vi "DAQ_Configure.vi"(8 "error in":errorcluster caption="entrée d'erreur", 10 "Dwell time (µs)":dbl, 11 "Scanning positions":dbl[][](array[numeric])) -> (0 "error out":errorcluster caption="sortie d'erreur", 3 "Task cluster":T1)   [LabVIEW 2026]
uses:
  <vilib>/DAQmx/write.llb/DAQmx Write (Analog 2D DBL NChan NSamp).vi
  <vilib>/DAQmx/create/channels.llb/DAQmx Create Channel (CO-Pulse Generation-Frequency).vi
  <vilib>/DAQmx/configure/timing.llb/DAQmx Timing (Implicit).vi
  <vilib>/DAQmx/create/channels.llb/DAQmx Create Channel (AO-Voltage-Basic).vi
  <vilib>/DAQmx/configure/timing.llb/DAQmx Timing (Sample Clock).vi
  <vilib>/DAQmx/miscellaneous.llb/DAQmx Fill In Error Info.vi
  <vilib>/DAQmx/create/channels.llb/DAQmx Create Channel (AI-Voltage-Basic).vi
  <vilib>/DAQmx/configure/trigger.llb/DAQmx Start Trigger (Digital Edge).vi
  <vilib>/DAQmx/create/channels.llb/DAQmx Create Channel (CI-Pulse Width).vi
  <resource>/objmgr/daqmx.rc
panel:
  out "N samples":u16
  out "Pixel_Freq":dbl
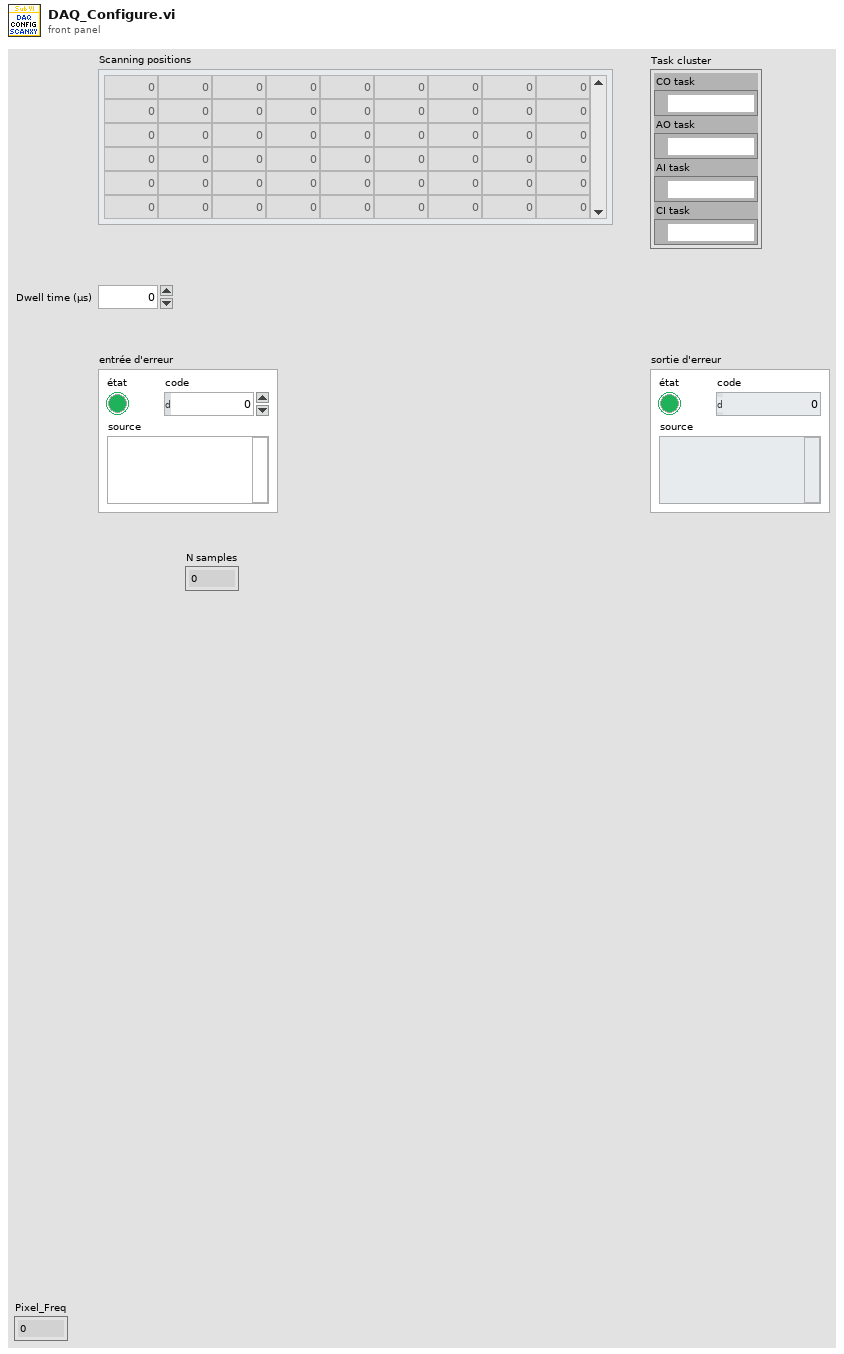
[diagram p1: front panel]
types:
  T1 = cluster{"CO task":refnum<k21>, "AO task":refnum<k21>, "AI task":refnum<k21>, "CI task":refnum<k21>}
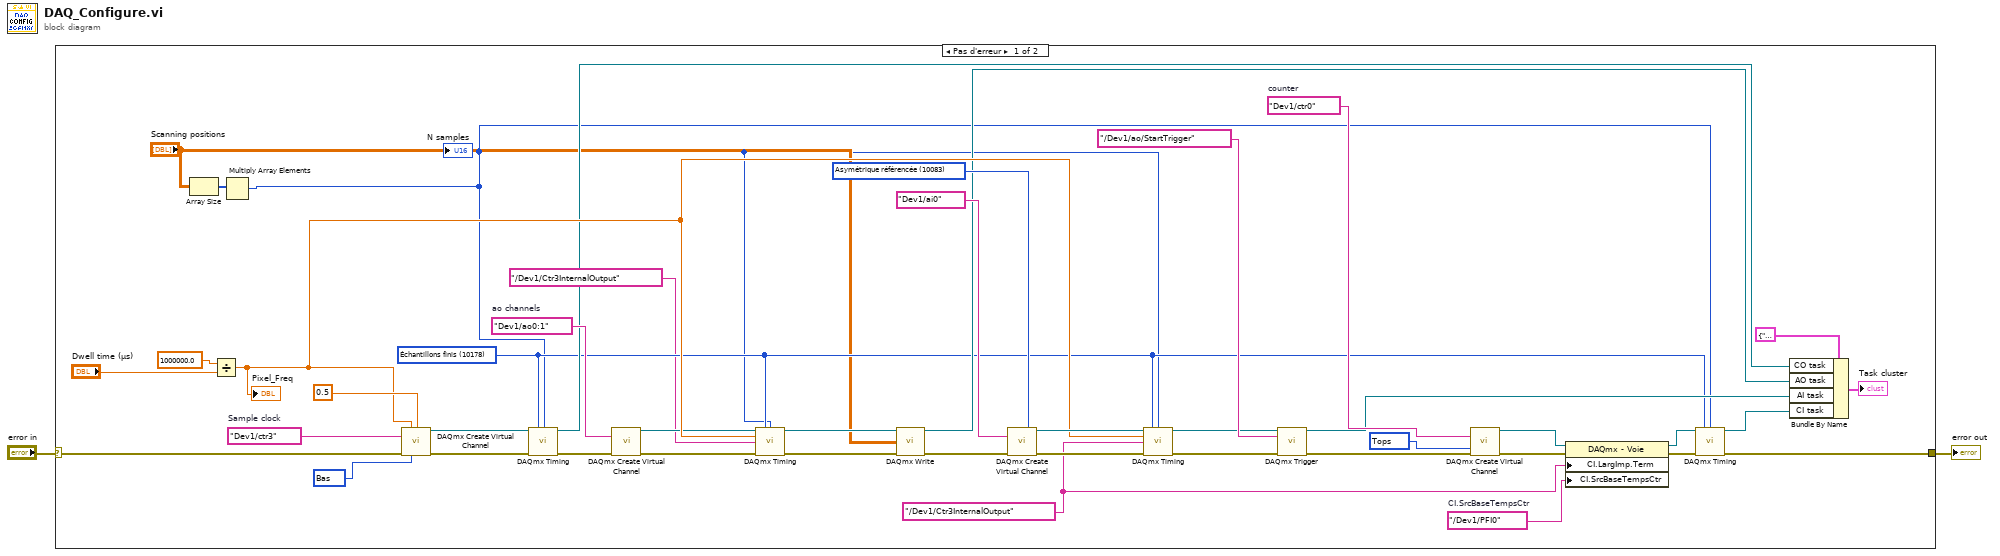
[diagram p0: block diagram]
diagram:
  n1 = case shown="Pas d'erreur" "error in" {
    selector: "error in" -> [w44 w47]
    tunnel: [w13 w47] -> w1
    frame No Error {
      w22 = tag "/Dev1/PFI0"  # CI.SrcBaseTempsCtr
      w28 = 10304 items=["Secondes"=10364, "Tops"=10304, "D'une échelle personnalisée"=10065] ("units")
      w29 = tag "Dev1/ctr0"  # counter
      w25 = tag "/Dev1/Ctr3InternalOutput" ("source")
      w35 = 10083 items=["Par défaut"=-1, "Asymétrique référencée"=10083, "Asymétrique non référencée"=10078, "Différentielle"=10106, "Pseudodifférentielle"=12529] ("input terminal configuration")
      w37 = tag "Dev1/ao0:1"  # ao channels
      w12 = 10178 items=["Échantillons finis"=10178, "Échantillons continus"=10123, "Point par point avec cadencement matériel"=12522] ("sample mode")
      w39 = 10214 items=["Haut"=10192, "Bas"=10214] ("idle state")
      w41 = tag "Dev1/ctr3"  # Sample clock
      n2 = Array Size(array="Scanning positions") -> (size(s)=w5:i32[])
      n3 = Divide(x=1000000.0, y="Dwell time (µs)") -> (x/y=w32:dbl)
      "Pixel_Freq" <- w32
      n4 = Multiply Array Elements(1:w5) -> (0:w3:i32)
      "N samples" <- w3
      n5 = call-poly <vilib>:"DAQmx Create Virtual Channel.vi"("frequency"=w32, "duty cycle"=0.5 ("Duty cycle"), "counter"=w41, "error in"=w44, "idle state"=w39) -> ("task out"=w43:refnum<k21>, "error out"=w42:errorcluster)  [unwired: 9 in]
      n6 = call-poly <vilib>:"DAQmx Timing.vi"("task/channels in"=w43, "sample mode"=w12, "samples per channel"=w3, "error in"=w42) -> ("task out"=w21:refnum<k21>, "error out"=w38:errorcluster)  [unwired: 10 in]
      n7 = call-poly <vilib>:"DAQmx Create Virtual Channel.vi"("physical channels"=w37, "error in"=w38) -> ("task out"=w10:refnum<k21>, "error out"=w11:errorcluster)  [unwired: 12 in]
      n8 = call-poly <vilib>:"DAQmx Timing.vi"("task/channels in"=w10, "sample mode"=w12, "samples per channel"=w3, "rate"=w32, "source"=tag "/Dev1/Ctr3InternalOutput", "error in"=w11) -> ("task out"=w8:refnum<k21>, "error out"=w7:errorcluster)  [unwired: 8 in]
      n9 = call-poly <vilib>:"DAQmx Write.vi"("task/channels in"=w8, "data"="Scanning positions", "error in"=w7) -> ("task out"=w18:refnum<k21>, "error out"=w30:errorcluster)  [unwired: 10 in, 1 out]
      n10 = call-poly <vilib>:"DAQmx Create Virtual Channel.vi"("input terminal configuration"=w35, "physical channels"=tag "Dev1/ai0", "error in"=w30) -> ("task out"=w34:refnum<k21>, "error out"=w33:errorcluster)  [unwired: 11 in]
      n11 = call-poly <vilib>:"DAQmx Timing.vi"("task/channels in"=w34, "sample mode"=w12, "samples per channel"=w3, "rate"=w32, "source"=w25, "error in"=w33) -> ("task out"=w16:refnum<k21>, "error out"=w15:errorcluster)  [unwired: 8 in]
      n12 = call-poly <vilib>:"DAQmx Trigger.vi"("task/channels in"=w16, "source"=tag "/Dev1/ao/StartTrigger", "error in"=w15) -> ("task out"=w17:refnum<k21>, "error out"=w6:errorcluster)  [unwired: 11 in]
      n13 = call-poly <vilib>:"DAQmx Create Virtual Channel.vi"("counter"=w29, "units"=w28, "error in"=w6) -> ("task out"=w26:refnum<k21>, "error out"=w27:errorcluster)  [unwired: 11 in]
      n14 = property class="DAQmx - Voie"(reference=w26, error in=w27, "CI.LargImp.Term"=w25, "CI.SrcBaseTempsCtr"=w22) -> (reference out=w24:refnum<k21>, error out=w23:errorcluster)
      n15 = call-poly <vilib>:"DAQmx Timing.vi"("task/channels in"=w24, "sample mode"=w12, "samples per channel"=w3, "error in"=w23) -> ("task out"=w14:refnum<k21>, "error out"=w13:errorcluster)  [unwired: 10 in]
      n16 = Bundle By Name(cluster=T1 {"CO task"="", "AO task"="", "AI task"="", "CI task"=""} ("cluster d'entrée"), "CO task"=w21, "AO task"=w18, "AI task"=w17, "CI task"=w14) -> (→"Task cluster":T1)
    }
    frame Error {
    }
  }
  "error out" <- w1
